vi "Cleanup.vi"(7 "Save (T)":bool, 8 "error in (no error)":errorcluster, 11 "PrefsDB in":refnum<class "PrefsDB.lvclass">) -> (0 "error out":errorcluster)   [LabVIEW 2020, in "User Prefs.lvlib" / "PrefsDB.lvclass"]
uses:
  PrefsDB.lvclass
  PrefsDB.lvclass/PrefsDB.ctl
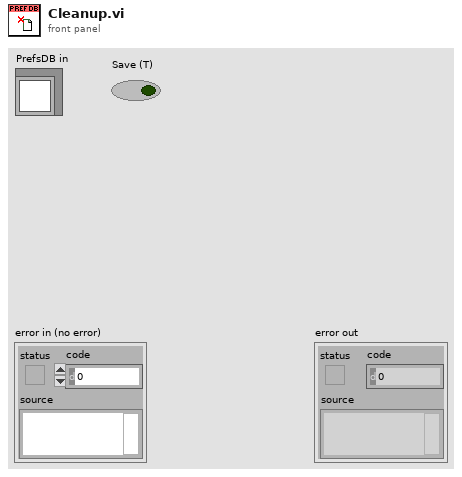
[diagram p1: front panel]
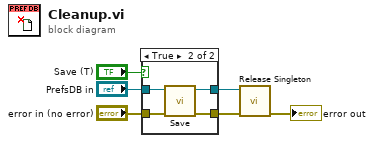
[diagram p0: block diagram]
diagram:
  n1 = case shown="True" "Save (T)" {
    tunnel: "PrefsDB in" -> [w8 w12]
    tunnel: "error in (no error)" -> [w7 w11]
    tunnel: [w7 w10] -> w3
    tunnel: [w8 w9] -> w1
    frame False {
    }
    frame True {
      n2 = call "Save.vi"("error in (no error)"=w11, "PrefsDB in"=w12) -> ("error out"=w10:errorcluster, "PrefsDB out"=w9:refnum<class "PrefsDB.lvclass">)  [unwired: 8 in]
    }
  }
  n3 = call "Release Singleton.vi"("error in (no error)"=w3, "PrefsDB in"=w1) -> ("error out"=→"error out":errorcluster)  [unwired: 9 in]
